vi "Get Crafting Stations.vi"(8 "error in (no error)":errorcluster, 11 "Blueprint in":refnum<class "Blueprint.lvclass">) -> (0 "error out":errorcluster, 2 "Stations":T1[](array[typedef]), 3 "Blueprint out":refnum<class "Blueprint.lvclass">)   [LabVIEW 2020, in "Blueprint.lvclass"]
uses:
  Blueprint.lvclass
  Item/Craft Station.ctl
  Workstation/Workstation.lvclass
  Assembly Table/Assembly Table.lvclass
  C:/dev/IlluminatedG/lv-oopanel-gc-calc/Workstation/Workstation.lvclass
  Blueprint.lvclass/Blueprint.ctl
  Item/Item.lvclass
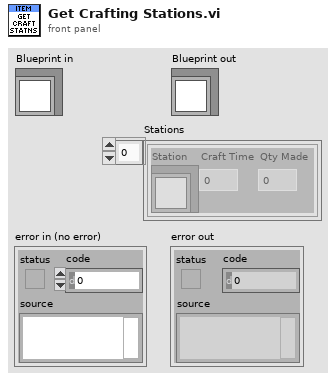
[diagram p1: front panel]
types:
  T1 = typedef "Item.lvclass/Craft Station.ctl" = cluster{"Station":refnum<class "Workstation.lvclass">, "Craft Time":dbl, "Qty Made":dbl}
  T2 = typedef "Blueprint.lvclass/Ref Data.ctl" = cluster{"Ingredients":T3[], "Workstation":refnum<class "Workstation.lvclass">, "Craft Time":dbl, "Name":string}
  T3 = typedef "Item.lvclass/Ingredient.ctl" = cluster{"Item":refnum<class "Item.lvclass">, "Qty":dbl}
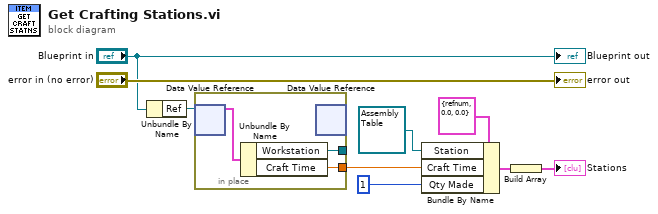
[diagram p0: block diagram]
diagram:
  n1 = Unbundle By Name("Blueprint in") -> ("Ref"=w8:refnum<data-value>)
  n2 = in-place {
    in-place-border: [w11] -> _
    in-place-border: [w10] -> w5
    n3 = in-place-dvr #1(w8) -> (w12:T2)  [unwired: 1 out]
    n4 = Unbundle By Name(w12) -> ("Workstation"=w11:refnum<class "Workstation.lvclass">, "Craft Time"=w10:dbl)
    n5 = in-place-dvr #1() -> ()  [unwired: 1 in, 2 out]
  }
  n6 = Bundle By Name(cluster=T1 {"Station"=refnum, "Craft Time"=0.0, "Qty Made"=0.0} ("Craft Station"), "Station"=refnum<class "Assembly Table.lvclass"> refnum ("Assembly Table.lvclass"), "Craft Time"=w5, "Qty Made"=1) -> (w4:T1)
  n7 = Build Array(w4) -> (→"Stations":T1[])
  "error out" <- "error in (no error)"
  "Blueprint out" <- "Blueprint in"
